vi "Scan for Hardware.vi"(8 "error in (no error)":errorcluster, 11 "Common Measurements in":refnum<class "Common Measurements.lvclass">) -> (0 "error out":errorcluster, 3 "Common Measurements out":refnum<class "Common Measurements.lvclass">)   [LabVIEW 2015, in "Common Measurements.lvclass"]
uses:
  Common Measurements.lvclass
  Mag Lab Measure Controller/Mag Lab Measure Controller.lvclass
  Mag Lab Measure Base/Mag Lab Measure Base.lvclass
  Mag Lab Error Handler/Mag Lab Error Handler.lvclass
  Mag Lab Root/Mag Lab Root.lvclass
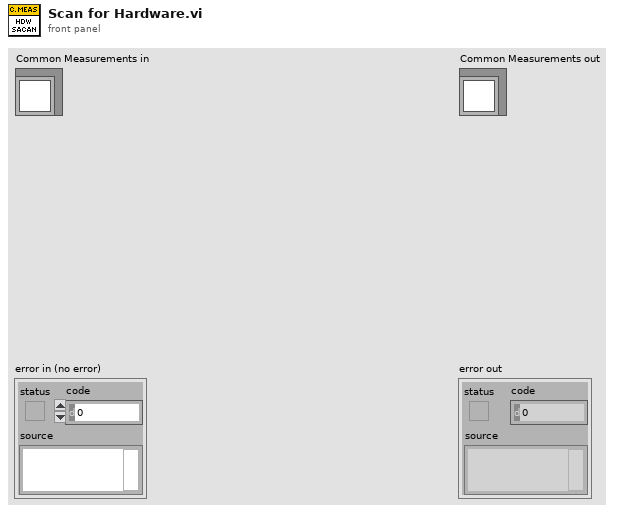
[diagram p1: front panel]
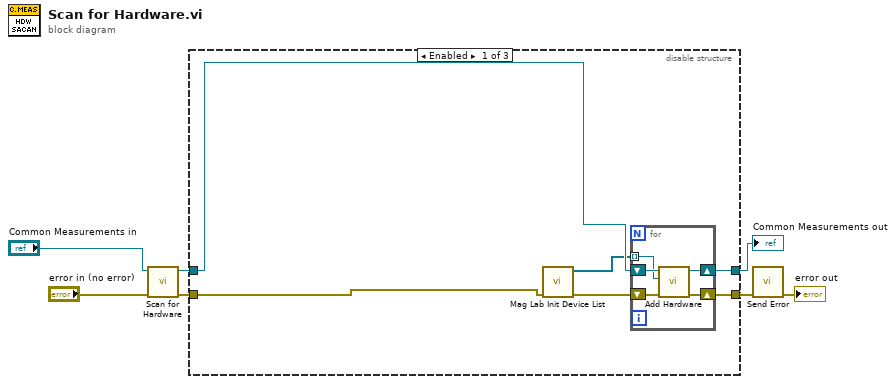
[diagram p0: block diagram]
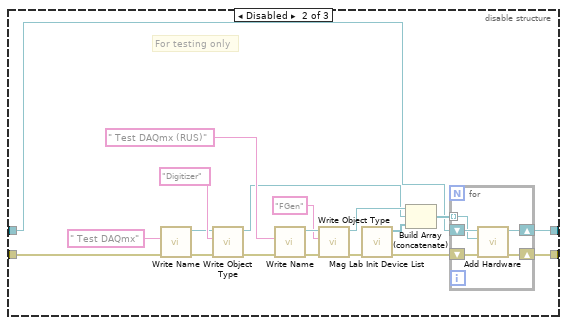
[diagram p2: hidden frame]
diagram:
  n1 = call-parent "Scan for Hardware.vi"("error in (no error)"="error in (no error)", "Mag Lab Measure Controller in"="Common Measurements in") -> ("error out"=w5:errorcluster, "Mag Lab Measure Controller out"=w4:refnum<class "Common Measurements.lvclass">)  [unwired: 8 in]
  n2 = disable-structure shown="Enabled" {
    disable-tunnel: w5 -> [w9 w32 w45]
    disable-tunnel: w4 -> [w13 w27 w46]
    disable-tunnel: [w12 w26 w46] -> w3
    disable-tunnel: [w11 w25 w45] -> w2
    frame Enabled {
      n3 = call "Mag Lab Init Device List.vi"("error in (no error)"=w9) -> ("error out"=w10:errorcluster, "Found Array"=w8:refnum<class "Mag Lab Hardware.lvclass">[])  [unwired: 8 in, 1 out]
      n4 = for {
        shift-right: [w17] -> w12
        shift-left: w13 -> [w18]
        tunnel: w8 -> [w16] mode=indexing
        shift-right: [w14] -> w11
        shift-left: w10 -> [w15]
        n5 = call-dynamic "Add Hardware.vi"("error in (no error)"=w15, "Mag Lab Hardware.lvclass"=w16, "Mag Lab Measure Controller in"=w18) -> ("error out"=w14:errorcluster, "Mag Lab Measure Controller out"=w17:refnum<class "Common Measurements.lvclass">)  [unwired: 7 in]
      }
    }
    frame Disabled {
      # "For testing only"
      n6 = call "Write Name.vi"("error in (no error)"=w32, "Name"=" Test DAQmx" ("string")) -> ("error out"=w23:errorcluster, "Mag Lab Root out"=w22:refnum<class "Mag Lab Root.lvclass">, "Mag Lab Root in"=w33:refnum<class "Mag Lab Root.lvclass">)  [unwired: 7 in]
      n7 = call "Write Object Type.vi"("error in (no error)"=w23, "Object Type"="Digitizer", "Mag Lab Measure Base in"=w22) -> ("error out"=w31:errorcluster, "Mag Lab Measure Base out"=w29:refnum<class "Mag Lab Measure Base.lvclass">)  [unwired: 7 in]
      n8 = call "Write Name.vi"("error in (no error)"=w31, "Name"=" Test DAQmx (RUS)" ("string")) -> ("error out"=w38:errorcluster, "Mag Lab Root out"=w39:refnum<class "Mag Lab Root.lvclass">, "Mag Lab Root in"=w36:refnum<class "Mag Lab Root.lvclass">)  [unwired: 7 in]
      n9 = call "Write Object Type.vi"("error in (no error)"=w38, "Object Type"="FGen", "Mag Lab Measure Base in"=w39) -> ("error out"=w21:errorcluster, "Mag Lab Measure Base out"=w30:refnum<class "Mag Lab Measure Base.lvclass">)  [unwired: 7 in]
      n10 = call "Mag Lab Init Device List.vi"("error in (no error)"=w21) -> ("error out"=w20:errorcluster, "Found Array"=w19:refnum<class "Mag Lab Hardware.lvclass">[])  [unwired: 8 in, 1 out]
      n11 = Build Array (concatenate)(w30, w29, w19) -> (w28:refnum<class "Mag Lab Measure Base.lvclass">[])
      n12 = for {
        shift-right: [w43] -> w26
        shift-left: w27 -> [w44]
        tunnel: w28 -> [w42] mode=indexing
        shift-right: [w40] -> w25
        shift-left: w20 -> [w41]
        n13 = call-dynamic "Add Hardware.vi"("error in (no error)"=w41, "Mag Lab Hardware.lvclass"=w42, "Mag Lab Measure Controller in"=w44) -> ("error out"=w40:errorcluster, "Mag Lab Measure Controller out"=w43:refnum<class "Common Measurements.lvclass">)  [unwired: 7 in]
      }
    }
    frame Disabled {
    }
  }
  "Common Measurements out" <- w3
  n14 = call "Send Error.vi"("error in (no error)"=w2) -> ("error out"=→"error out":errorcluster)  [unwired: 9 in, 1 out]
